vi "Get Node Text Content.vi"(8 "error in (no error)":errorcluster, 11 "node in":refnum<k20>) -> (0 "error out":errorcluster, 2 "node text":string, 3 "node out":refnum<k20>)   [LabVIEW 2018, in "NI_XML.lvlib"]
doc: "Returns the combined values of <B>Text_Node</B> children that the <B>node in</B> node owns."
uses:
  NI_XML.lvlib
  Close Reference(Node).vi
  C:/Program Files (x86)/National Instruments/LabVIEW 2018/resource/objmgr/DOMUserDefRef.rc
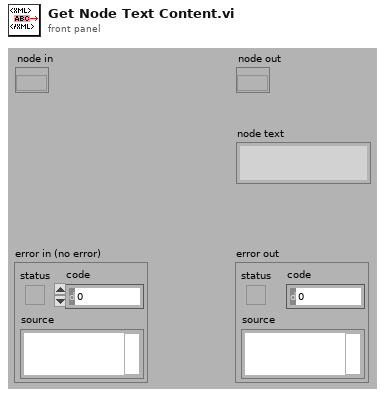
[diagram p1: front panel]
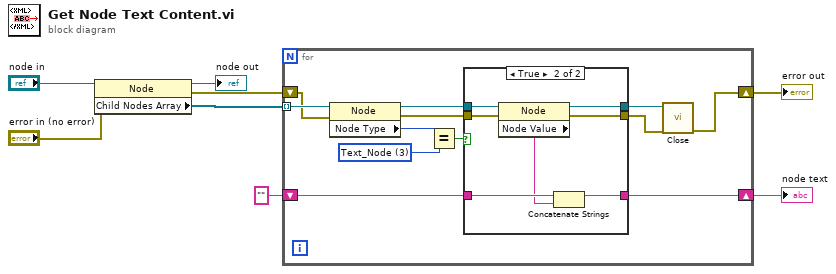
[diagram p0: block diagram]
diagram:
  n1 = property class="Node"(reference="node in", error in="error in (no error)") -> (reference out=→"node out":refnum<k20>, error out=w6:errorcluster, "Child Nodes Array"=w5:refnum<k20>[])
  n2 = for {
    shift-right: [w10] -> w2
    shift-left: w6 -> [w19]
    tunnel: w5 -> [w20] mode=indexing
    shift-right: [w9] -> w1
    shift-left: "" -> [w13]
    w17 = 3 items=["Element_Node"=1, "Attribute_Node"=2, "Text_Node"=3, "CDATASection_Node"=4, "EntityReference_Node"=5, "Entity_Node"=6, "ProcessingInstruction_Node"=7, "Comment_Node"=8, "Document_Node"=9, "DocumentType_Node"=10, "DocumentFragment_Node"=11, "Notation_Node"=12] ("Node Type")
    n3 = property class="Node"(reference=w20, error in=w19) -> (reference out=w15:refnum<k20>, error out=w14:errorcluster, "Node Type"=w18:i32)
    n4 = Equal?(x=w18, y=w17) -> (x = y?=w16:bool)
    n5 = case shown="True" w16 {
      tunnel: w15 -> [w22 w30]
      tunnel: w14 -> [w21 w29]
      tunnel: w13 -> [w23 w28]
      tunnel: [w23 w26] -> w9
      tunnel: [w22 w25] -> w12
      tunnel: [w21 w24] -> w11
      frame False {
      }
      frame True {
        n6 = property class="Node"(reference=w30, error in=w29) -> (reference out=w25:refnum<k20>, error out=w24:errorcluster, "Node Value"=w27:string)
        n7 = Concatenate Strings(w28, w27) -> (w26:string)
      }
    }
    n8 = call-poly "Close.vi"("error in (no error)"=w11, "node"=w12) -> ("error out"=w10:errorcluster)  [unwired: 7 out]
  }
  "error out" <- w2
  "node text" <- w1
